vi "hModeReg2014.vi"(4 "error in":errorcluster, 5 "Range":u8, 6 "Mode":u16 format="%x", 7 "FPGA VI Reference In":refnum<k20>) -> (0 "error out":errorcluster, 2 "Timeout":bool, 3 "FPGA VI Reference Out":refnum<k20>)   [LabVIEW 2014]
doc: "Schreibt eine gemeinsame Konfiguration in alle Moderegister."
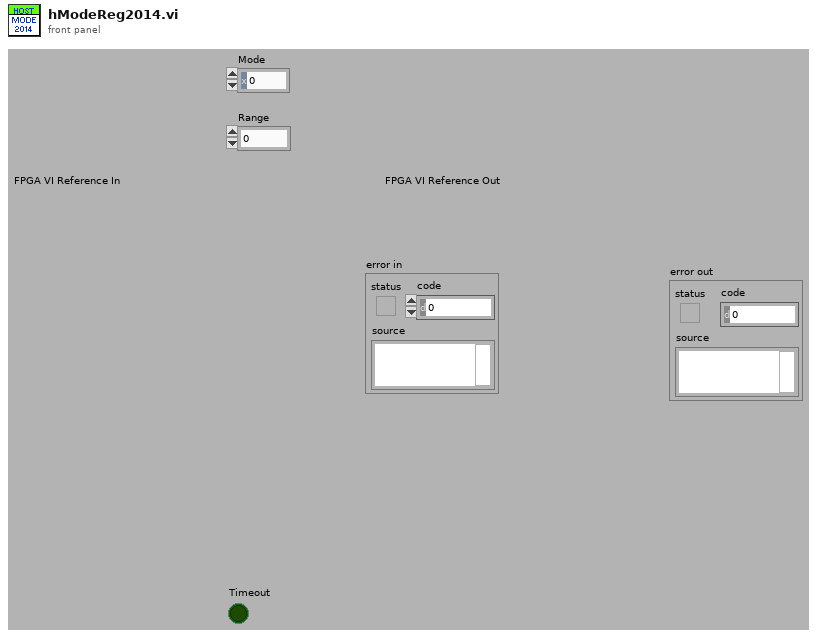
[diagram p1: front panel]
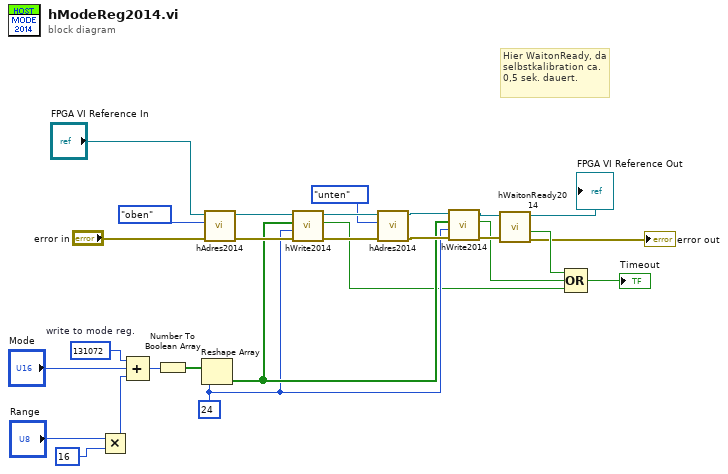
[diagram p0: block diagram]
diagram:
  w25 = u32 131072  # write to mode reg.
  w9 = u8 24
  # "Hier WaitonReady, da selbstkalibration ca. 0,5 sek. dauert."
  n1 = Multiply(x="Range", y=u8 16) -> (x*y=w23:u8)
  n2 = Compound Arithmetic op=unknown(w25, "Mode", w23) -> (w26:u32)
  n3 = Number To Boolean Array(number=w26) -> (Boolean array=w24:bool[])
  n4 = Reshape Array(w24, w9) -> (w10:bool[])
  n5 = call "hAdres2014.vi"("error in"="error in", "AdressMode"=enum16{"select", "oben", "unten", "keinen"}."oben", "FPGA VI Reference In"="FPGA VI Reference In") -> ("error out"=w13:errorcluster, "FPGA VI Reference Out"=w18:refnum<k20>)  [unwired: 3 in]
  n6 = call "hWrite2014.vi"("error in"=w13, "nbit"=w9, "Data"=w10, "FPGA VI Reference In"=w18) -> ("error out"=w14:errorcluster, "Timed Out"=w2:bool, "FPGA VI Reference Out"=w19:refnum<k20>)  [unwired: 1 in]
  n7 = call "hAdres2014.vi"("error in"=w14, "AdressMode"=enum16{"select", "oben", "unten", "keinen"}."unten", "FPGA VI Reference In"=w19) -> ("error out"=w11:errorcluster, "FPGA VI Reference Out"=w12:refnum<k20>)  [unwired: 3 in]
  n8 = call "hWrite2014.vi"("error in"=w11, "nbit"=w9, "Data"=w10, "FPGA VI Reference In"=w12) -> ("error out"=w8:errorcluster, "Timed Out"=w3:bool, "FPGA VI Reference Out"=w7:refnum<k20>)  [unwired: 1 in]
  n9 = call "hWaitonReady2014.vi"("error in"=w8, "FPGA VI Reference In"=w7) -> ("error out"=→"error out":errorcluster, "Timeout"=w6:bool, "FPGA VI Reference Out"=→"FPGA VI Reference Out":refnum<k20>)  [unwired: 3 in]
  n10 = Compound Arithmetic op=OR(w6, w3, w2) -> (→"Timeout":bool)
